vi "read_ini.vi"(11 "Path_bench":path) -> (1 "value":i64)   [LabVIEW 2014]
uses:
  <vilib>/Utility/config.llb/Read Key (I32).vi
  <vilib>/Utility/config.llb/NI_LVConfig.lvlib
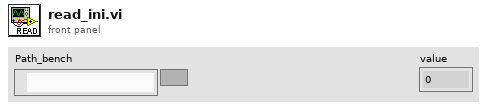
[diagram p1: front panel]
types:
  T1 = typedef "NI_LVConfig.lvlib/Config Data RefNum.ctl" = refnum<k1>
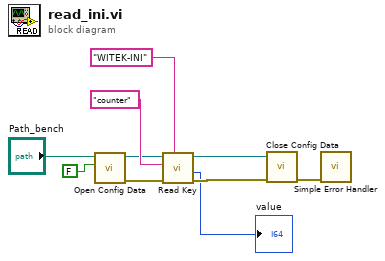
[diagram p0: block diagram]
diagram:
  n1 = call <vilib>:"Open Config Data.vi"("create file if necessary (T)"=FALSE, "configuration file path"="Path_bench") -> ("error out"=w9:errorcluster, "refnum"=w7:T1)  [unwired: 7 in, 1 out]
  n2 = call-poly <vilib>:"Read Key.vi"("section"="WITEK-INI", "error in (no error)"=w9, "key"="counter", "refnum"=w7) -> ("error out"=w6:errorcluster, "value"=→"value":i32, "refnum out"=w5:T1)  [unwired: 4 in, 1 out]
  n3 = call <vilib>:"Close Config Data.vi"("error in (no error)"=w6, "refnum"=w5) -> ("error out"=w4:errorcluster)  [unwired: 8 in, 1 out]
  n4 = call <vilib>:"Simple Error Handler.vi"("error in (no error)"=w4) -> ()  [unwired: 4 in, 5 out]
